vi "Climb.vi"() -> ()   [LabVIEW 2015]
uses:
  Common Code/Climb Status in Auto.ctl
  Common Code/Climb Manual Controls.ctl
  Robot Global Data.vi
panel:
  out "Boolean 5":bool=TRUE
  out "Boolean 4":bool=TRUE
  out "Boolean 3":bool=TRUE
  out "Boolean 1":bool=TRUE
  out "Boolean":bool=TRUE
  in  "Numeric":dbl
  in  "PTO Controls":T1
  in  "Manual Sequence":T2
  in  "Mode Auto":T3
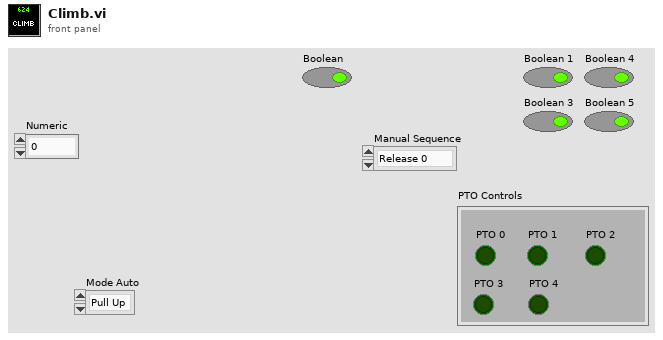
[diagram p1: front panel]
types:
  T1 = cluster{"PTO 0":bool, "PTO 1":bool, "PTO 2":bool, "PTO 3":bool, "PTO 4":bool}
  T2 = typedef "Climb Manual Controls.ctl" = enum16{"Release 0", "Release 1", "Winch Begin"}
  T3 = typedef "Climb Status in Auto.ctl" = enum16{"Pull Up", "Hold On", "Reach Up"}
  T4 = typedef "Climb Mode.ctl" = enum16{"Auto", "Manual"}
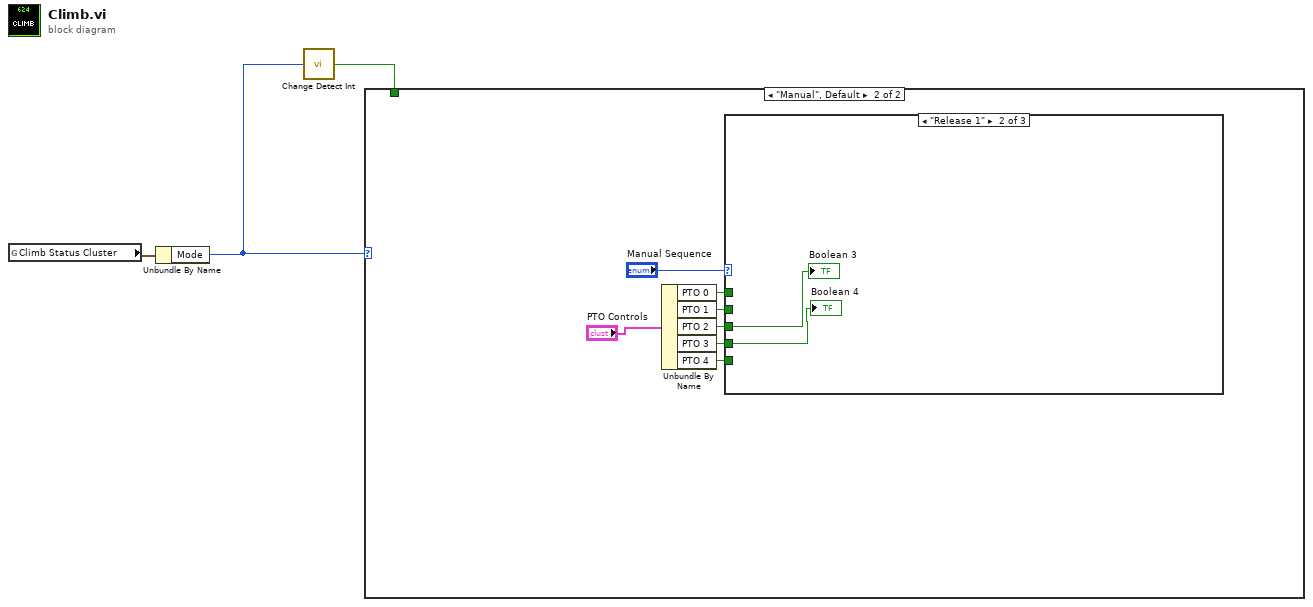
[diagram p0: block diagram]
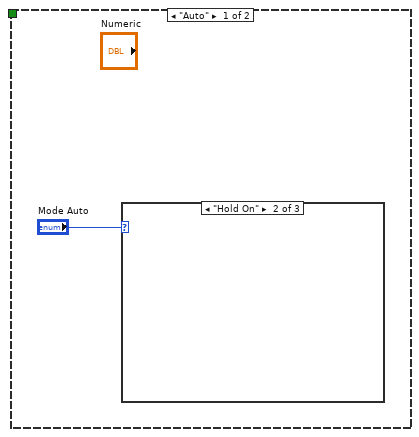
[diagram p2: hidden frame]
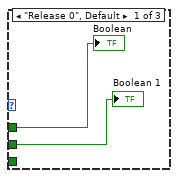
[diagram p5: hidden frame]
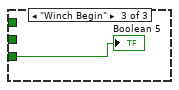
[diagram p6: hidden frame]
diagram:
  n1 = global read "Robot Global Data.vi" "Climb Status Cluster"() -> (w3:cluster{"Mode":T4})
  n2 = Unbundle By Name(w3) -> ("Mode"=w2:T4)
  n3 = call "Change Detect Int.vi"("In"=w2) -> ("Changed?"=w1:bool)
  n4 = case shown="\"Manual\", Default" w2 {
    tunnel: w1 -> [_ _]
    frame "Auto" {
      n5 = case shown="\"Hold On\"" "Mode Auto" {
        frame "Pull Up", Default {
        }
        frame "Hold On" {
        }
        frame "Reach Up" {
        }
      }
    }
    frame "Manual", Default {
      n6 = Unbundle By Name("PTO Controls") -> ("PTO 0"=w9:bool, "PTO 1"=w8:bool, "PTO 2"=w7:bool, "PTO 3"=w6:bool, "PTO 4"=w5:bool)
      n7 = case shown="\"Release 1\"" "Manual Sequence" {
        tunnel: w9 -> [w13 _ _]
        tunnel: w8 -> [w12 _ _]
        tunnel: w7 -> [_ w15 _]
        tunnel: w6 -> [_ w14 _]
        tunnel: w5 -> [_ _ w16]
        frame "Release 0", Default {
          "Boolean" <- w13
          "Boolean 1" <- w12
        }
        frame "Release 1" {
          "Boolean 3" <- w15
          "Boolean 4" <- w14
        }
        frame "Winch Begin" {
          "Boolean 5" <- w16
        }
      }
    }
  }
